vi "cc1.vi"() -> ()   [LabVIEW 2020]
uses:
  LabVIEW Example(8.6)/ControlCAN/ControlCAN.lvlib
  LabVIEW Example(8.6)/ControlCAN/ControlCAN.llb/DevType.ctl
  LabVIEW Example(8.6)/ControlCAN/ControlCAN.llb/VCI_CAN_OBJ.ctl
  TEST1/ControlCAN/ControlCAN.llb/InitFlag.ctl
  TEST1/ControlCAN/ControlCAN.llb/Fliter.ctl
  TEST1/ControlCAN/ControlCAN.llb/Mode.ctl
  TEST1/ControlCAN/ControlCAN.llb/VCI_INIT_CONFIG.ctl
  LabVIEW Example(8.6)/ControlCAN/ControlCAN.llb/Return Val.ctl
panel:
  in  "Data[4] 2":u8
  in  "Data[4]":u8
  in  "设定速度":i16
  out "波形图表":dbl(graph)
  in  "停止":bool
  in  "READ":bool
  out "实际速度":i16
  out "Return Val 2":T1=1 items=["OK"=1, "ERROR1"=0, "ERROR2"=-1]
  out "Recieve[0].Data":u8[](array[numeric])
  out "Recieve":T2[](array[typedef])
  in  "Len":u32=2500 caption="Len(2500)"
  out "Recieve 2":T2[](array[typedef])
  out "子字符串":string
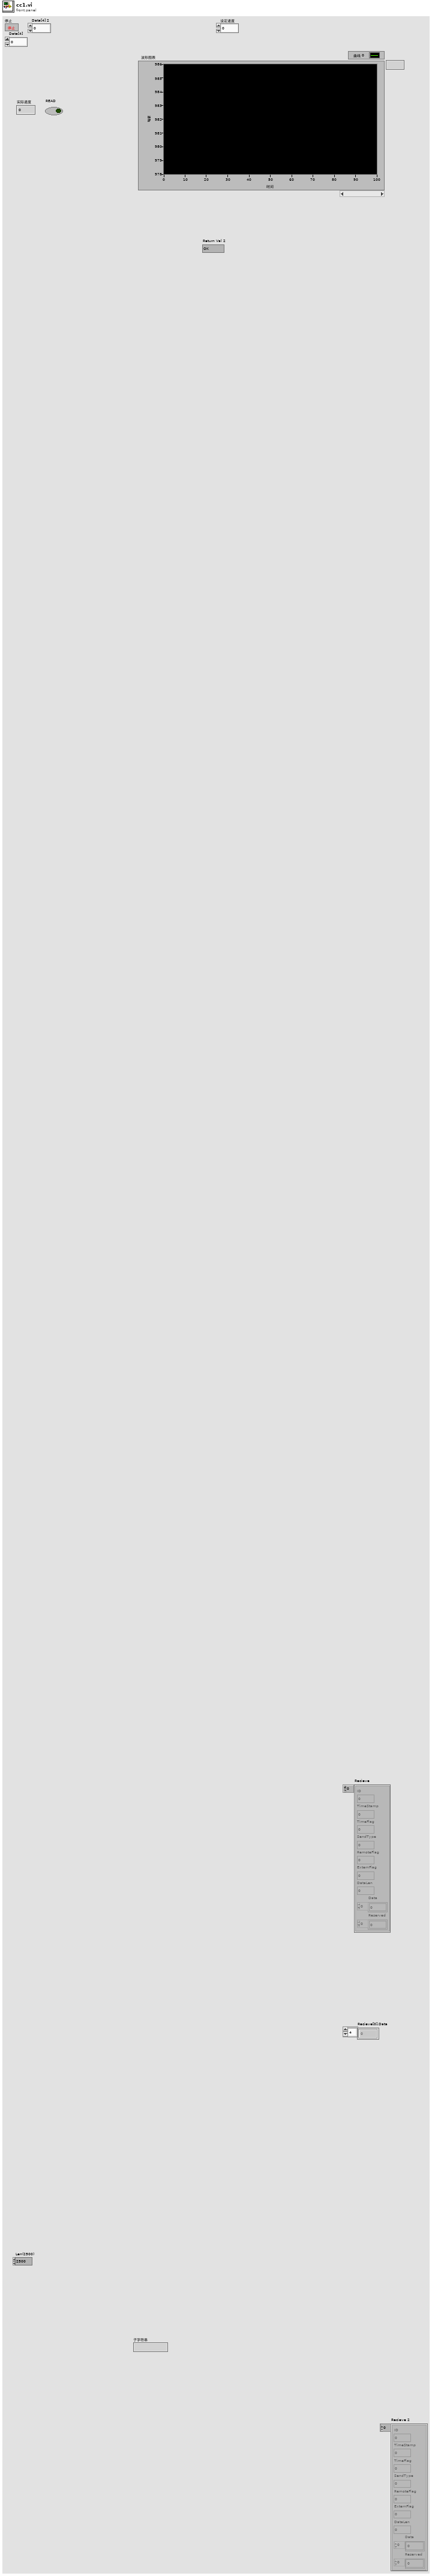
[diagram p1: front panel]
types:
  T1 = typedef "ControlCAN.lvlib/Return Val.ctl" = i32
  T2 = typedef "ControlCAN.lvlib/VCI_CAN_OBJ.ctl" = cluster{"ID":u32, "TimeStamp":u32, "TimeFlag":u8, "SendType":u8, "RemoteFlag":u8, "ExternFlag":u8, "DataLen":u8, "Data":u8[], "Reserved":u8[]}
  T3 = typedef "ControlCAN.lvlib/VCI_INIT_CONFIG.ctl" = cluster{"AccCode":u32, "AccMask":u32, "InitFlag":T4, "Fliter":T5, "Timing0":u8, "Timing1":u8, "Mode":T6}
  T4 = typedef "ControlCAN.lvlib/InitFlag.ctl" = u32
  T5 = typedef "ControlCAN.lvlib/Fliter.ctl" = u8
  T6 = typedef "ControlCAN.lvlib/Mode.ctl" = u8
  T7 = typedef "ControlCAN.lvlib/DevType.ctl" = u32
  T8 = cluster{"Recieve[0]":T2, "Recieve[1]":T2, "Recieve[2]":T2, "Recieve[3]":T2, "Recieve[4]":T2, "Recieve[5]":T2, "Recieve[6]":T2, "Recieve[7]":T2, "Recieve[8]":T2}
  T9 = cluster{"Data[0]":u8, "Data[1]":u8, "Data[2]":u8, "Data[3]":u8, "Data[4]":u8, "Data[5]":u8, "Data[6]":u8, "Data[7]":u8, "Data[8]":u8}
  T10 = cluster{"Buffer[0]":T2, "Buffer[1]":T2, "Buffer[2]":T2, "Buffer[3]":T2, "Buffer[4]":T2, "Buffer[5]":T2, "Buffer[6]":T2, "Buffer[7]":T2, "Buffer[8]":T2}
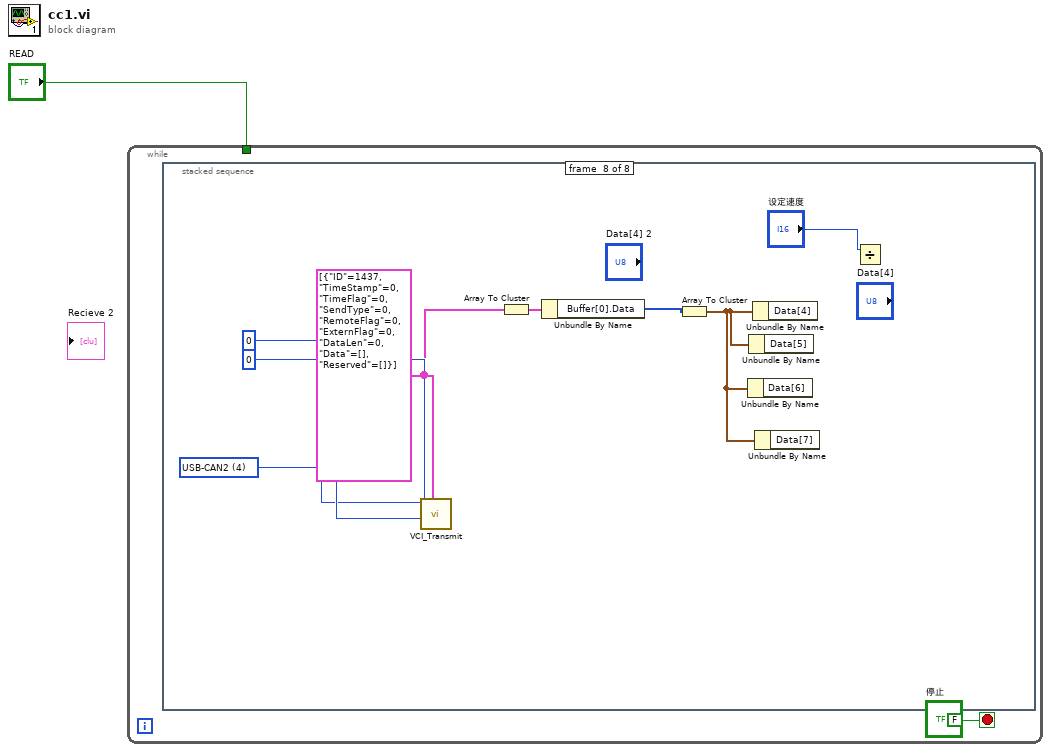
[diagram p0: block diagram]
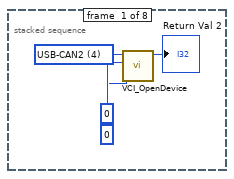
[diagram p2: hidden frame]
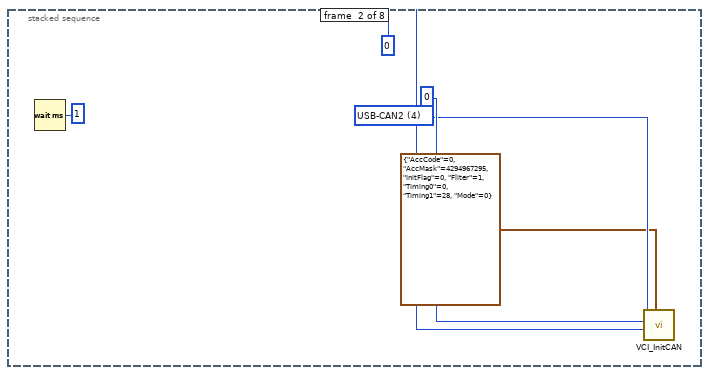
[diagram p3: hidden frame]
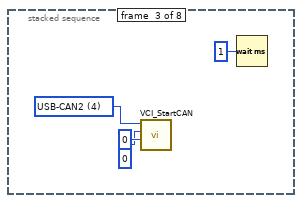
[diagram p4: hidden frame]
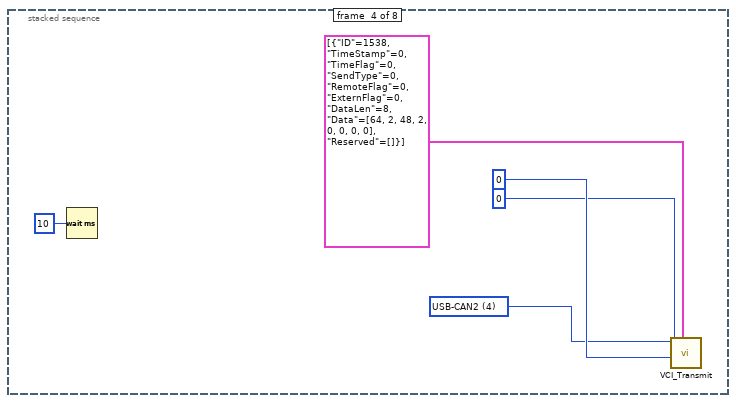
[diagram p5: hidden frame]
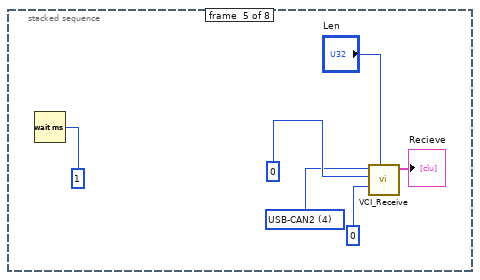
[diagram p6: hidden frame]
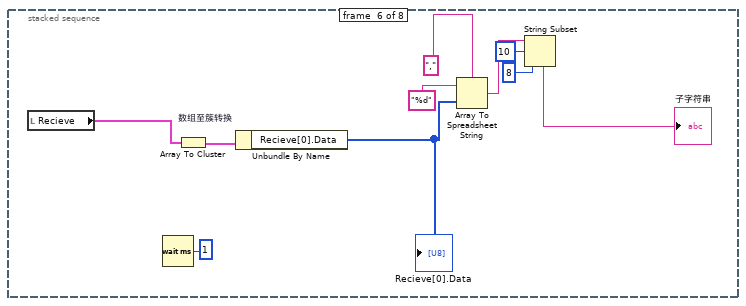
[diagram p7: hidden frame]
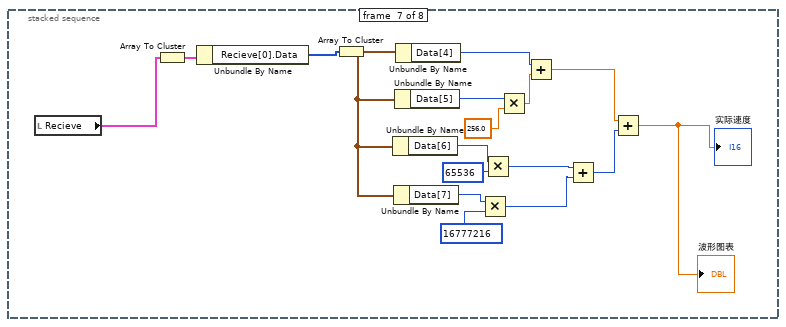
[diagram p8: hidden frame]
diagram:
  n1 = while {
    tunnel: "READ" -> [_]
    stop <- FALSE stop-if-true
    n2 = stacked-sequence {
      frame #0 {
        w3 = T7 4 items=["USB-CAN"=3, "USB-CAN2"=4] ("DevType")
        n3 = call "VCI_OpenDevice.vi"("Reserved"=u32 0, "DevIndex"=u32 0, "DevType"=w3) -> ("Return Val"=→"Return Val 2":T1)  [unwired: 7 in, 1 out]
      }
      frame #1 {
        w9 = T7 4 items=["USB-CAN"=3, "USB-CAN2"=4] ("DevType")
        n4 = Wait (ms)(milliseconds to wait=u32 1 ("等待时间（毫秒）")) -> ()  [unwired: 1 out]
        n5 = call "VCI_InitCAN.vi"("VCI_INIT_CONFIG"=T3 {"AccCode"=0, "AccMask"=4294967295, "InitFlag"=0, "Fliter"=1, "Timing0"=0, "Timing1"=28, "Mode"=0}, "CANIndex"=u32 0, "DevIndex"=u32 0, "DevType"=w9) -> ()  [unwired: 6 in, 2 out]
      }
      frame #2 {
        w13 = T7 4 items=["USB-CAN"=3, "USB-CAN2"=4] ("DevType")
        n6 = call "VCI_StartCAN.vi"("CANIndex"=u32 0, "DevIndex"=u32 0, "DevType"=w13) -> ()  [unwired: 7 in, 2 out]
        n7 = Wait (ms)(milliseconds to wait=u32 1 ("等待时间（毫秒）")) -> ()  [unwired: 1 out]
      }
      frame #3 {
        w17 = T7 4 items=["USB-CAN"=3, "USB-CAN2"=4] ("DevType")
        n8 = Wait (ms)(milliseconds to wait=u32 10 ("等待时间（毫秒）")) -> ()  [unwired: 1 out]
        n9 = call "VCI_Transmit.vi"("Buffer"=T2[] [{"ID"=1538, "TimeStamp"=0, "TimeFlag"=0, "SendType"=0, "RemoteFlag"=0, "ExternFlag"=0, "DataLen"=8, "Data"=[64, 2, 48, 2, 0, 0, 0, 0], "Reserved"=[]}], "CANIndex"=u32 0, "DevIndex"=u32 0, "DevType"=w17) -> ()  [unwired: 6 in, 2 out]
      }
      frame #4 {
        w21 = T7 4 items=["USB-CAN"=3, "USB-CAN2"=4] ("DevType")
        n10 = Wait (ms)(milliseconds to wait=u32 1 ("等待时间（毫秒）")) -> ()  [unwired: 1 out]
        n11 = call "VCI_Receive.vi"("Len"="Len", "CANIndex"=u32 0, "DevIndex"=u32 0, "DevType"=w21) -> ("Recieve"=→"Recieve":T2[])  [unwired: 6 in, 1 out]
      }
      frame #5 {
        n12 = local read "Recieve"() -> (w36:T2[])
        n13 = Wait (ms)(milliseconds to wait=u32 1 ("等待时间（毫秒）")) -> ()  [unwired: 1 out]
        n14 = Array To Cluster "数组至簇转换"(array=w36) -> (cluster=w29:T8)
        n15 = Unbundle By Name(w29) -> ("Recieve[0].Data"=w31:u8[])
        "Recieve[0].Data" <- w31
        n16 = Array To Spreadsheet String(delimiter (Tab)="," ("分隔符(Tab)"), array=w31, 3:"%d" ("格式字符串")) -> (spreadsheet string=w33:string)
        n17 = String Subset(string=w33, offset (0)=10 ("偏移量(0)"), length (rest)=8 ("长度（剩余）")) -> (substring=→"子字符串":string)
      }
      frame #6 {
        n18 = local read "Recieve"() -> (w53:T2[])
        n19 = Array To Cluster(array=w53) -> (cluster=w52:T8)
        n20 = Unbundle By Name(w52) -> ("Recieve[0].Data"=w51:u8[])
        n21 = Array To Cluster(array=w51) -> (cluster=w50:T9)
        n22 = Unbundle By Name(w50) -> ("Data[6]"=w45:u8)
        n23 = Unbundle By Name(w50) -> ("Data[7]"=w44:u8)
        n24 = Unbundle By Name(w50) -> ("Data[5]"=w49:u8)
        n25 = Unbundle By Name(w50) -> ("Data[4]"=w46:u8)
        n26 = Multiply(x=w44, y=16777216) -> (x*y=w40:i32)
        n27 = Multiply(x=w45, y=65536) -> (x*y=w41:i32)
        n28 = Multiply(x=w49, y=256.0) -> (x*y=w47:dbl)
        n29 = Add(x=w46, y=w47) -> (x+y=w39:dbl)
        n30 = Add(x=w41, y=w40) -> (x+y=w38:i32)
        n31 = Add(x=w39, y=w38) -> (x+y=→"实际速度" →"波形图表":dbl)
      }
      frame #7 {
        w58 = T2[] [{"ID"=1437, "TimeStamp"=0, "TimeFlag"=0, "SendType"=0, "RemoteFlag"=0, "ExternFlag"=0, "DataLen"=0, "Data"=[], "Reserved"=[]}] ("Buffer")
        w59 = T7 4 items=["USB-CAN"=3, "USB-CAN2"=4] ("DevType")
        n32 = call "VCI_Transmit.vi"("Buffer"=w58, "CANIndex"=u32 0, "DevIndex"=u32 0, "DevType"=w59) -> ()  [unwired: 6 in, 2 out]
        n33 = Array To Cluster(array=w58) -> (cluster=w57:T10)
        n34 = Unbundle By Name(w57) -> ("Buffer[0].Data"=w56:u8[])
        n35 = Array To Cluster(array=w56) -> (cluster=w55:T9)
        n36 = Unbundle By Name(w55) -> ()  [unwired: 1 out]
        n37 = Unbundle By Name(w55) -> ()  [unwired: 1 out]
        n38 = Unbundle By Name(w55) -> ()  [unwired: 1 out]
        n39 = Unbundle By Name(w55) -> ()  [unwired: 1 out]
        n40 = Divide(x="设定速度") -> ()  [unwired: 1 in, 1 out]
      }
    }
  }
